vi "4峰值多周期平均子程序.vi"(1 "波形":waveform(dbl)) -> (0 "f":dbl)   [LabVIEW 2017]
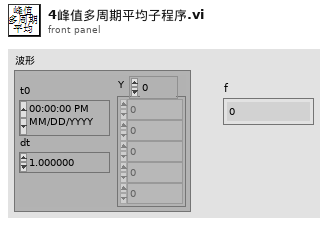
[diagram p1: front panel]
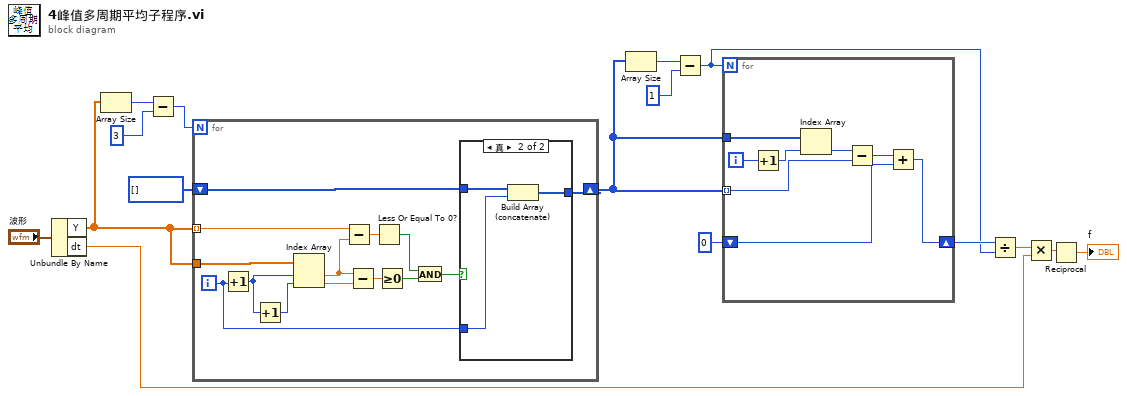
[diagram p0: block diagram]
diagram:
  n1 = Unbundle By Name("波形") -> ("Y"=w7:dbl[], "dt"=w13:dbl)
  n2 = Array Size(array=w7) -> (size(s)=w6:i32)
  n3 = Subtract(x=w6, y=3) -> (x-y=w4:i32)
  n4 = for {
    N: w4 -> [_]
    tunnel: w7 -> [w21] mode=indexing
    tunnel: w7 -> [w30]
    shift-right: [w24] -> w10
    shift-left: i32[] [] -> [w25]
    i -> [w26]
    n5 = Increment(x=w26) -> (x+1=w23:i32)
    n6 = Increment(x=w23) -> (x+1=w22:i32)
    n7 = Index Array(array=w30, index #1=w23, index #2=w22) -> (element #1=w19:dbl, element #2=w17:dbl)
    n8 = Subtract(x=w21, y=w19) -> (x-y=w20:dbl)
    n9 = Subtract(x=w19, y=w17) -> (x-y=w18:dbl)
    n10 = Less Or Equal To 0?(x=w20) -> (x <= 0?=w28:bool)
    n11 = Greater Or Equal To 0?(x=w18) -> (x >= 0?=w29:bool)
    n12 = And(x=w28, y=w29) -> (x .and. y?=w27:bool)
    n13 = case shown="真" w27 {
      tunnel: w26 -> [_ w34]
      tunnel: w25 -> [w31 w32]
      tunnel: [w31 w33] -> w24
      frame False {
      }
      frame True {
        n14 = Build Array (concatenate)(w32, w34) -> (w33:i32[])
      }
    }
  }
  n15 = Array Size(array=w10) -> (size(s)=w3:i32)
  n16 = Subtract(x=w3, y=1) -> (x-y=w1:i32)
  n17 = for {
    N: w1 -> [_]
    tunnel: w10 -> [w38] mode=indexing
    tunnel: w10 -> [w42]
    shift-right: [w35] -> w9
    shift-left: 0 -> [w36]
    i -> [w41]
    n18 = Increment(x=w41) -> (x+1=w40:i32)
    n19 = Index Array(array=w42, index=w40) -> (element=w39:i32)
    n20 = Subtract(x=w39, y=w38) -> (x-y=w37:i32)
    n21 = Add(x=w37, y=w36) -> (x+y=w35:i32)
  }
  n22 = Divide(x=w9, y=w1) -> (x/y=w8:dbl)
  n23 = Multiply(x=w8, y=w13) -> (x*y=w12:dbl)
  n24 = Reciprocal(x=w12) -> (1/x=→"f":dbl)
